vi "Queue INI TCP and NT Table Stream Queue.vi"() -> (3 "Queue out":refnum<queue>)   [LabVIEW 2025]
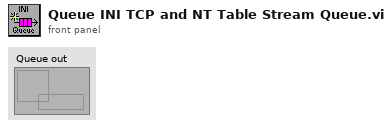
[diagram p1: front panel]
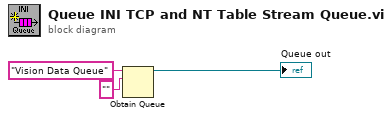
[diagram p0: block diagram]
diagram:
  n1 = Obtain Queue(name (unnamed)="Vision Data Queue", element data type="" ("concatenated string")) -> (queue out=→"Queue out":refnum<queue>)  [unwired: 3 in, 2 out]
